vi "DiffDriveOdom_Trajectory_SetAuto.vi"(11 "Ramsete AUTO":bool) -> ()   [LabVIEW 2019]
uses:
  DiffDriveOdom_Trajectory_Globals.vi
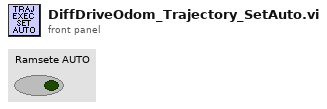
[diagram p1: front panel]
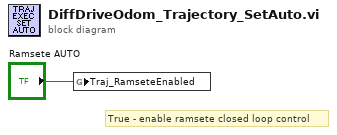
[diagram p0: block diagram]
diagram:
  # "True - enable ramsete closed loop control"
  n1 = global write "DiffDriveOdom_Trajectory_Globals.vi" "Traj_RamseteEnabled"("Ramsete AUTO") -> ()
